vi "Append.datIfReqd.vi"(11 "Path":path) -> (3 "appended path":path)   [LabVIEW 2013]
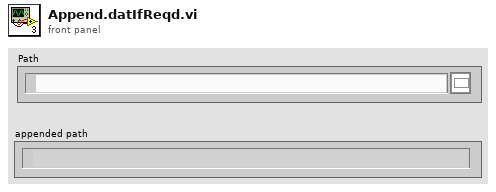
[diagram p1: front panel]
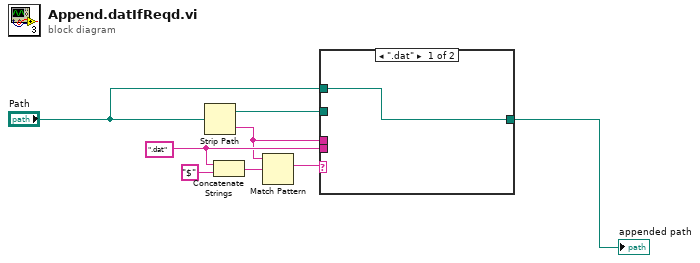
[diagram p0: block diagram]
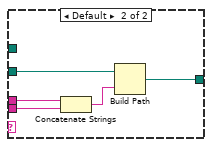
[diagram p2: hidden frame]
diagram:
  w6 = ".dat" ("string")
  n1 = Strip Path(path="Path") -> (stripped path=w3:path, name=w4:string)
  n2 = Concatenate Strings(w6, "$" ("string")) -> (w5:string)
  n3 = Match Pattern(string=w4, regular expression=w5) -> (match substring=w8:string)  [unwired: 1 in, 3 out]
  n4 = case shown="\".dat\"" w8 {
    tunnel: [w9 w14] -> w2
    tunnel: w3 -> [_ w13]
    tunnel: w4 -> [_ w11]
    tunnel: w6 -> [_ w10]
    tunnel: "Path" -> [w9 _]
    frame ".dat" {
    }
    frame Default {
      n5 = Concatenate Strings(w11, w10) -> (w12:string)
      n6 = Build Path(base path=w13, name or relative path=w12) -> (appended path=w14:path)
    }
  }
  "appended path" <- w2
